vi "Get Classes Names.vi"() -> (3 "Classes":string[](array[string]))   [LabVIEW 2020]
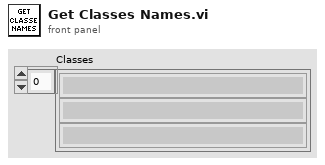
[diagram p1: front panel]
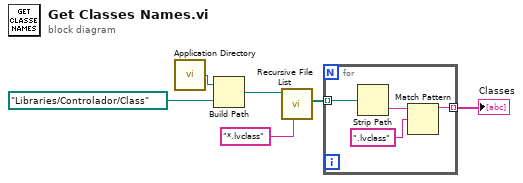
[diagram p0: block diagram]
diagram:
  n1 = call <vilib>:"Application Directory.vi"() -> ("Application Directory"=w5:path)
  n2 = Build Path(base path=w5, name or relative path=path "Libraries/Controlador/Class") -> (appended path=w4:path)
  n3 = call <vilib>:"Recursive File List.vi"("pattern"="*.lvclass", "Folder Path"=w4) -> ("All Files in Dir"=w1:path[])  [unwired: 5 in, 4 out]
  n4 = for {
    tunnel: w1 -> [w8] mode=indexing
    tunnel: [w7] -> w3 mode=indexing
    n5 = Strip Path(path=w8) -> (name=w9:string)  [unwired: 1 out]
    n6 = Match Pattern(string=w9, regular expression=".lvclass") -> (before substring=w7:string)  [unwired: 1 in, 3 out]
  }
  "Classes" <- w3
